vi "EnumerateAPI.vi"(8 "error in (no error)":errorcluster, 11 "Node in":refnum<class "PyObject.lvclass">) -> (0 "error out":errorcluster, 2 "API":string[](array[string]), 3 "Node out":refnum<class "PyObject.lvclass">)   [LabVIEW 2013, in "JKI_Python_Bridge_for_LV.lvlib" / "PyObject.lvclass"]
uses:
  PyObject.lvclass
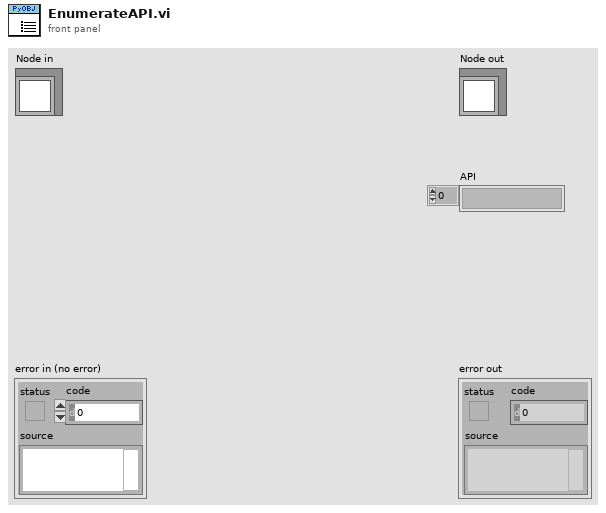
[diagram p1: front panel]
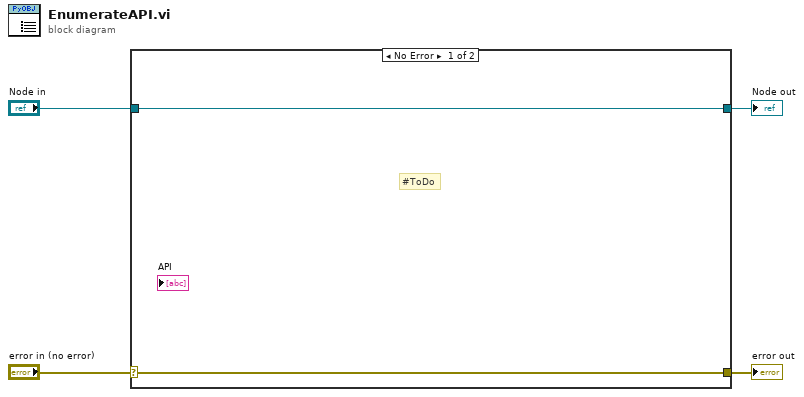
[diagram p0: block diagram]
diagram:
  n1 = case shown="No Error" "error in (no error)" {
    selector: "error in (no error)" -> [w5 w8]
    tunnel: [w5 w8] -> w3
    tunnel: [w6 w7] -> w1
    tunnel: "Node in" -> [w6 w7]
    frame No Error {
      # "#ToDo"
    }
    frame Error {
    }
  }
  "error out" <- w3
  "Node out" <- w1
